vi "getLastData.vi"(7 "LabVIEW Web Service Request":refnum<class "Web Request.lvclass">) -> ()   [LabVIEW 2016]
uses:
  <vilib>/wsapi/Web Request.lvclass
  Typedef/Device data.ctl
  <vilib>/Utility/file.llb/Read Delimited Spreadsheet (string).vi
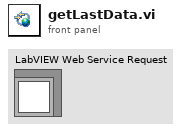
[diagram p1: front panel]
types:
  T1 = typedef "Device data.ctl" = cluster{"MAC Address":string, "Label":string, "Data":dbl[][]}
  T2 = enum16{"open", "replace", "create", "open or create", "replace or create", "replace or create with confirmation"}
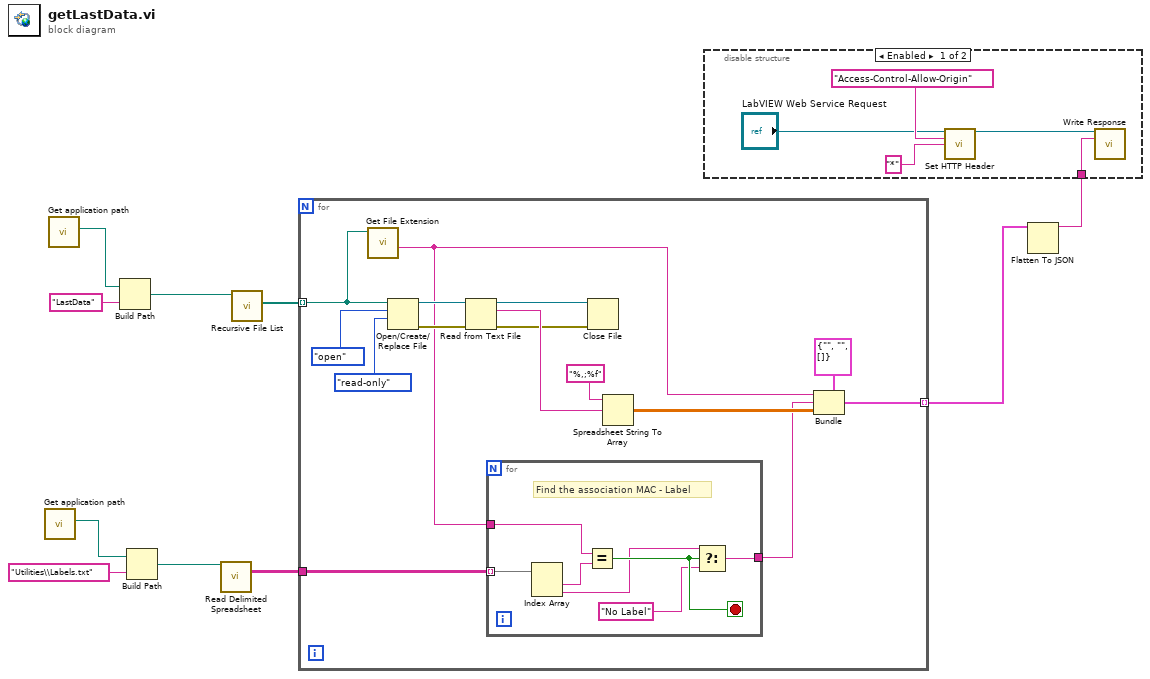
[diagram p0: block diagram]
diagram:
  n1 = call "Get application path.vi"() -> ("Application path"=w1:path)  [unwired: 11 in]
  n2 = call "Get application path.vi"() -> ("Application path"=w2:path)  [unwired: 11 in]
  n3 = Build Path(base path=w2, name or relative path="LastData") -> (appended path=w10:path)
  n4 = Build Path(base path=w1, name or relative path="Utilities\\Labels.txt") -> (appended path=w6:path)
  n5 = call-poly <vilib>:"Read Delimited Spreadsheet.vi"("file path (dialog if empty)"=w6) -> ("all rows"=w5:string[][])  [unwired: 9 in, 5 out]
  n6 = call <vilib>:"Recursive File List.vi"("Folder Path"=w10) -> ("All Files in Dir"=w9:path[])  [unwired: 6 in, 4 out]
  n7 = for {
    tunnel: w9 -> [w17] mode=indexing
    tunnel: [w16] -> w8 mode=indexing
    tunnel: w5 -> [w14]
    n8 = call <vilib>:"Get File Extension.vi"("file"=w17) -> ("filename without extension"=w13:string)  [unwired: 6 in, 4 out]
    n9 = Open/Create/Replace File(file path (use dialog)=w17, operation (0:open)=T2."open", access (0:read/write)=enum16{"read/write", "read-only", "write-only"}."read-only") -> (refnum out=w25:refnum<file>, error out=w24:errorcluster)  [unwired: 3 in, 1 out]
    n10 = Read from Text File(file (use dialog)=w25, error in=w24) -> (refnum out=w20:refnum<file>, text=w21:string, error out=w19:errorcluster)  [unwired: 2 in, 1 out]
    n11 = for {
      tunnel: w14 -> [w32] mode=indexing
      tunnel: w13 -> [w31]
      tunnel: [w28] -> w11
      stop <- w30 stop-if-true
      # "Find the association MAC - Label"
      n12 = Index Array(array=w32) -> (element #1=w27:string, element #2=w29:string)  [unwired: 2 in]
      n13 = Equal?(x=w31, y=w27) -> (x = y?=w30:bool)
      n14 = Select(t=w29, s=w30, f="No Label") -> (s? t:f=w28:string)
    }
    n15 = Close File(refnum=w20, error in=w19) -> ()  [unwired: 2 out]
    n16 = Spreadsheet String To Array(format string="%,;%f", spreadsheet string=w21) -> (array=w12:dbl[][])  [unwired: 2 in]
    n17 = Bundle(cluster=T1 {"MAC Address"="", "Label"="", "Data"=[]} ("Device data"), "MAC Address"=w13, "Label"=w11, "Data"=w12) -> (w16:T1)
  }
  n18 = Flatten To JSON(anything=w8) -> (JSON string=w7:string)  [unwired: 2 in, 1 out]
  n19 = disable-structure shown="Enabled" {
    disable-tunnel: w7 -> [w37 _]
    frame Enabled {
      n20 = call <vilib>:"Set HTTP Header.vi"("LabVIEW Web Service Request"="LabVIEW Web Service Request", "header"="Access-Control-Allow-Origin", "header value"="*") -> ("LabVIEW Web Service Request out"=w33:refnum<class "Web Request.lvclass">)  [unwired: 11 in, 1 out]
      n21 = call <vilib>:"Write Response.vi"("LabVIEW Web Service Request"=w33, "response string"=w37) -> ()  [unwired: 12 in, 2 out]
    }
    frame Disabled {
    }
  }
